vi "H5Oopen_by_idx.vi"(5 "Order":T1 items=["H5_ITER_UNKNOWN"=-1, "H5_ITER_INC"=0, "H5_ITER_DEC"=1], 6 "lapl_id":T3, 7 "Index Field":T2 items=["H5_INDEX_UNKNOWN"=-1, "H5_INDEX_NAME"=0, "H5_INDEX_CRT_ORDER"=1], 8 "error in (no error)":errorcluster, 9 "Index":u64, 10 "Name":string=".", 11 "Location Ref":T3) -> (0 "error out":errorcluster, 2 "Object Ref":T3, 3 "Location Ref out":T3)   [LabVIEW 2017]
doc: "Open the nth object in a group."
uses:
  <vilib>/UPVI/lvhdf5/library.llb/HDF5 Ref.ctl
  <vilib>/UPVI/lvhdf5/library.llb/H5_index_t.ctl
  <vilib>/UPVI/lvhdf5/library.llb/H5_iter_order_t.ctl
  <vilib>/UPVI/lvhdf5/hdf5.dll
panel:
  # "LVHDF5 Toolkit\nCopyright (c) 2005-2013 by Jason D. Sommerville\nCopyright (c) 2014-2015 by UPVI, LLC.\n\nThis use and distribution of this file is governed by the terms found in \nLICENSE.txt distributed with this toolkit and installed at\n <user.lib>\\_lvhdf5\\LICENSE.txt"
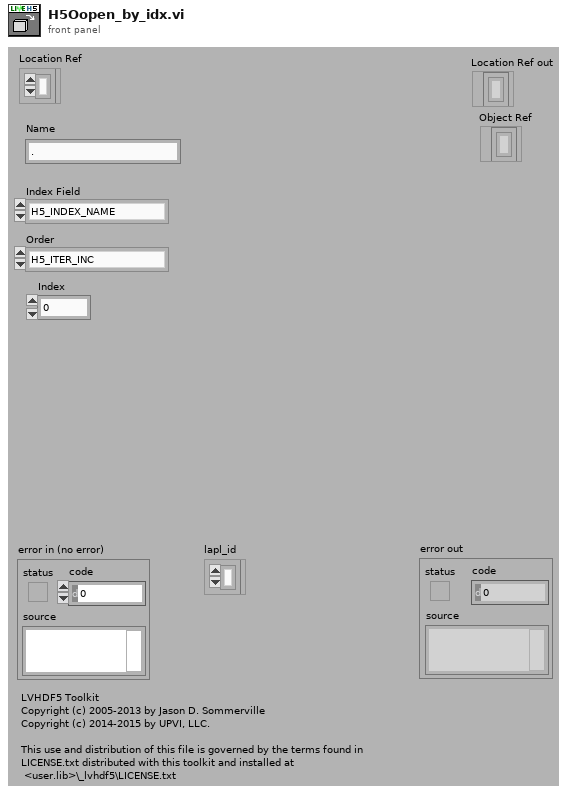
[diagram p1: front panel]
types:
  T1 = typedef "H5_iter_order_t.ctl" = i32
  T2 = typedef "H5_index_t.ctl" = i32
  T3 = typedef "HDF5 Ref.ctl" = refnum<k1>
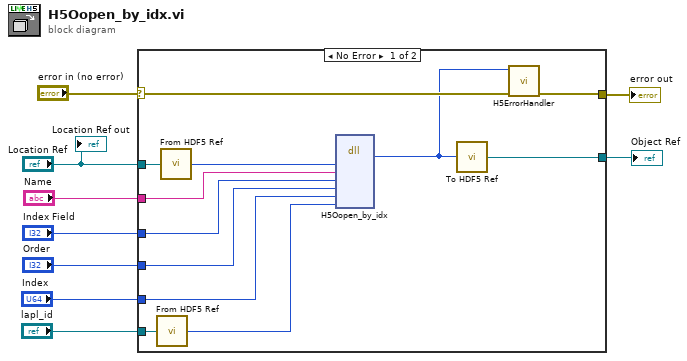
[diagram p0: block diagram]
diagram:
  n1 = case shown="No Error" "error in (no error)" {
    selector: "error in (no error)" -> [w21 w22]
    tunnel: [w20 w22] -> w8
    tunnel: "Location Ref" -> [w19 _]
    tunnel: "Name" -> [w17 _]
    tunnel: "lapl_id" -> [w16 _]
    tunnel: [w13 _] -> w4
    tunnel: "Index Field" -> [w12 _]
    tunnel: "Order" -> [w11 _]
    tunnel: "Index" -> [w10 _]
    frame No Error {
      n2 = call <vilib>:"From HDF5 Ref.vi"("HDF5 Ref"=w16) -> ("I32"=w15:i32)
      n3 = call <vilib>:"From HDF5 Ref.vi"("HDF5 Ref"=w19) -> ("I32"=w18:i32)
      n4 = dll-call lib="C:/Program Files/National Instruments/LabVIEW 2017/vi.lib/UPVI/lvhdf5/hdf5.dll" fn="H5Oopen_by_idx" label="H5Oopen_by_index"("loc_id"=w18, "name"=w17, "index_type"=w12, "order"=w11, "n"=w10, "lapl_id"=w15) -> ("return type"=w14:i32)  [unwired: 9 in, 2 out]
      n5 = call <vilib>:"To HDF5 Ref.vi"("I32"=w14) -> ("HDF5 Ref"=w13:T3)
      n6 = call <vilib>:"H5ErrorHandler.vi"("error in (no error)"=w21, "herr_t"=w14) -> ("error out"=w20:errorcluster)  [unwired: 3 in, 4 out]
    }
    frame Error {
    }
  }
  "error out" <- w8
  "Object Ref" <- w4
  "Location Ref out" <- "Location Ref"
